vi "Hardware - Use Optical Tracker.vi"(9 "Shared Variable Control":refnum<k21>="\\\\localhost\\SharedVariable\\EyeTrace", 10 "queue out":refnum<queue>, 11 "Waveforms in":waveform(dbl)[](array[waveform])) -> (3 "Waveforms out":waveform(dbl)[](array[waveform]))   [LabVIEW 2010]
uses:
  <vilib>/Analysis/NI_AALBase.lvlib
panel:
  in  "history":i32=3
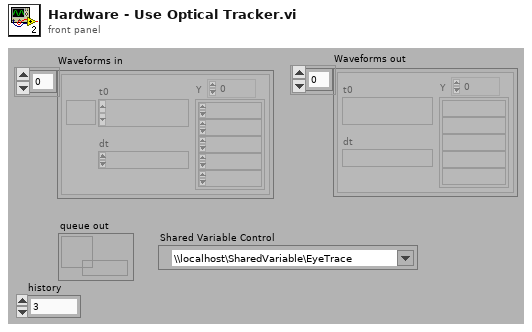
[diagram p1: front panel]
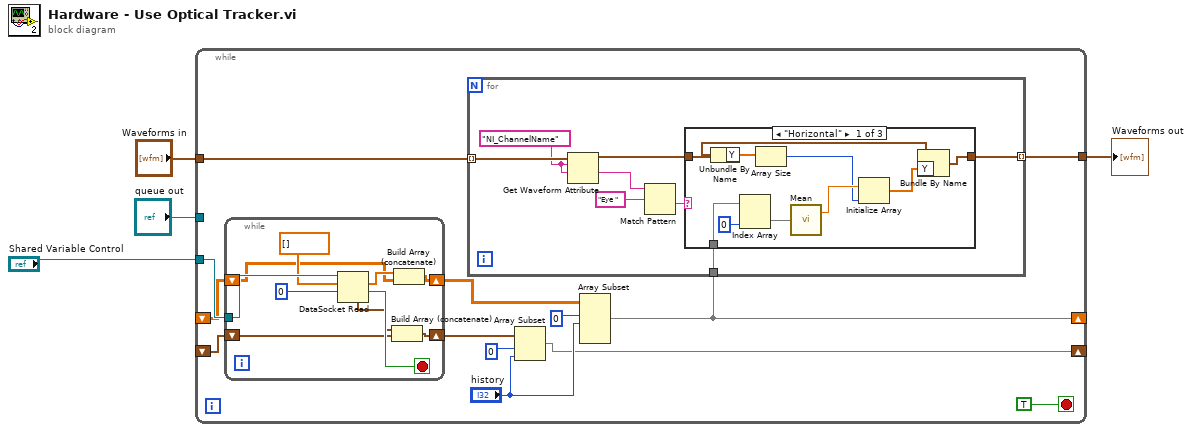
[diagram p0: block diagram]
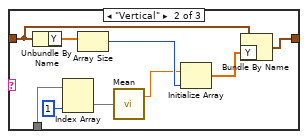
[diagram p2: hidden frame]
diagram:
  n1 = while {
    tunnel: "Waveforms in" -> [w17]
    tunnel: [w16] -> w3
    tunnel: "queue out" -> [_]
    shift-right: [w10] -> _
    shift-left: _ -> [w12]
    tunnel: "Shared Variable Control" -> [w13]
    shift-right: [w6] -> _
    shift-left: _ -> [w5]
    stop <- TRUE stop-if-true
    n2 = while {
      tunnel: w13 -> [w26]
      shift-right: [w21] -> w15
      shift-left: w12 -> [w22]
      shift-right: [w19] -> w8
      shift-left: w5 -> [w18]
      stop <- w24 stop-if-true
      n3 = DataSocket Read(9:0 ("ms timeout (10000)"), 10:dbl[] [], 11:w26) -> (1:w24:bool, 2:w23:dbl[], 4:w20:timestamp)  [unwired: 1 in, 5 out]
      n4 = Build Array (concatenate)(w20, w18) -> (w19:timestamp[])
      n5 = Build Array (concatenate)(w23, w22) -> (w21:dbl[][])
    }
    n6 = Array Subset(array=w8, index=0, length="history") -> (w6:timestamp[])
    n7 = Array Subset(array=w15, index (row)=0 ("index"), length (row)="history") -> (w10:dbl[][])  [unwired: 2 in]
    n8 = for {
      tunnel: w17 -> [w35] mode=indexing
      tunnel: [w29] -> w16 mode=indexing
      tunnel: w10 -> [w28]
      w32 = "NI_ChannelName" ("name")
      n9 = Get Waveform Attribute(5:w32, 6:w32, 7:w35) -> (1:w34:string, 3:w30:waveform(dbl))  [unwired: 1 in, 2 out]
      n10 = Match Pattern(string=w34, regular expression="Eye " ("values")) -> (after substring=w31:string)  [unwired: 4 out]
      n11 = case shown="\"Horizontal\"" w31 {
        tunnel: w30 -> [w43 w51 w54]
        tunnel: [w42 w50 w54] -> w29
        tunnel: w28 -> [w41 w53 _]
        frame "Horizontal" {
          n12 = Unbundle By Name(w43) -> ("Y"=w39:dbl[])
          n13 = Index Array(array=w41, index (col)=0 ("index (row)")) -> (element=w44:dbl[])  [unwired: 1 in]
          n14 = Array Size(array=w39) -> (size(s)=w38:i32)
          n15 = call <vilib>:"Mean.vi"("X"=w44) -> ("mean"=w40:dbl)  [unwired: 1 out]
          n16 = Initialize Array(w40, w38) -> (w37:dbl[])
          n17 = Bundle By Name(cluster=w43, "Y"=w37) -> (w42:waveform(dbl))
        }
        frame "Vertical" {
          n18 = Unbundle By Name(w51) -> ("Y"=w47:dbl[])
          n19 = Index Array(array=w53, index (col)=1 ("index (row)")) -> (element=w52:dbl[])  [unwired: 1 in]
          n20 = Array Size(array=w47) -> (size(s)=w49:i32)
          n21 = call <vilib>:"Mean.vi"("X"=w52) -> ("mean"=w48:dbl)  [unwired: 1 out]
          n22 = Initialize Array(w48, w49) -> (w46:dbl[])
          n23 = Bundle By Name(cluster=w51, "Y"=w46) -> (w50:waveform(dbl))
        }
        frame Default {
        }
      }
    }
  }
  "Waveforms out" <- w3
